vi "RT-Cert-Constants.vi"() -> (1 "Desired Repetitions":u32, 2 "Warmup Iterations":i32, 3 "Iterations":i32, 4 "Loop Period (us)":u32, 5 "CPU Cache":bool)   [LabVIEW 2014]
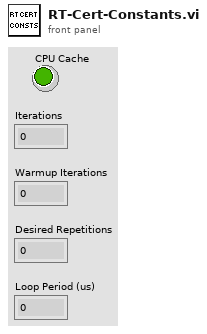
[diagram p1: front panel]
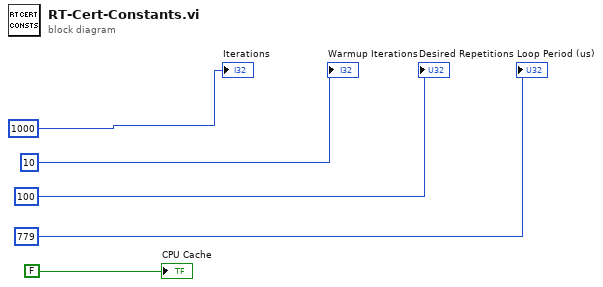
[diagram p0: block diagram]
diagram:
  "CPU Cache" <- FALSE ("CPU Cache")
  "Warmup Iterations" <- 10 ("Warmup Iterations")
  "Iterations" <- 1000 ("Iterations")
  "Desired Repetitions" <- u32 100 ("Desired Repetitions")
  "Loop Period (us)" <- u32 779 ("Loop Period (us)")
